vi "SearchAndReplaceString.vi"() -> ()   [LabVIEW 2019]
panel:
  out "OutputString":string
  in  "InputString":string
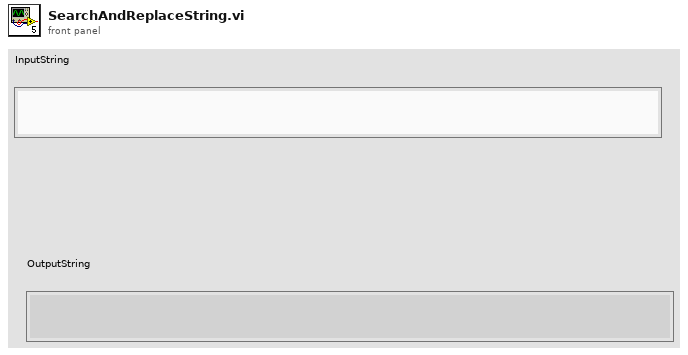
[diagram p1: front panel]
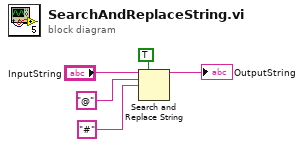
[diagram p0: block diagram]
diagram:
  n1 = Search and Replace String(replace all?=TRUE ("replace all? (F)"), input string="InputString", search string="@", replace string="#" ("search string")) -> (result string=→"OutputString":string)  [unwired: 4 in, 3 out]
